vi "Read Menu Queue.vi"(8 "error in (no error)":errorcluster, 11 "Interface with menu in":refnum<class "Interface with menu.lvclass">) -> (0 "error out":errorcluster, 2 "Actor Framework.lvlib:Message Enqueuer":refnum<class "Message Enqueuer.lvclass">, 3 "Interface with menu out":refnum<class "Interface with menu.lvclass">)   [LabVIEW 2015, in "Interface with menu.lvclass"]
uses:
  Interface with menu.lvclass
  <vilib>/ActorFramework/Message Enqueuer/Message Enqueuer.lvclass
  Interface with menu.lvclass/Interface with menu.ctl
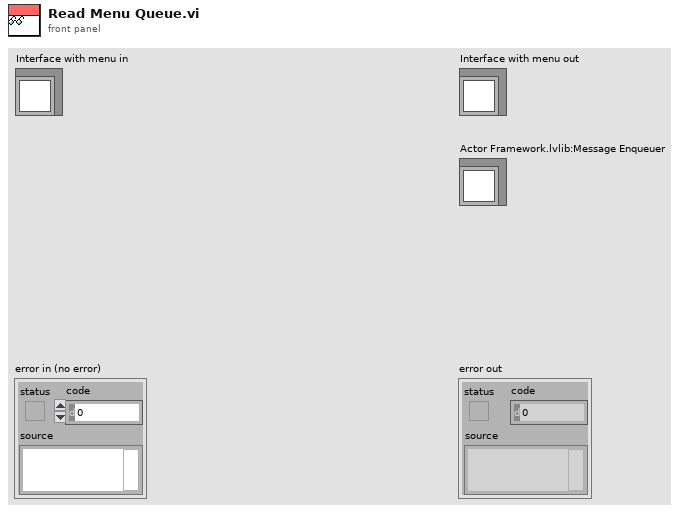
[diagram p1: front panel]
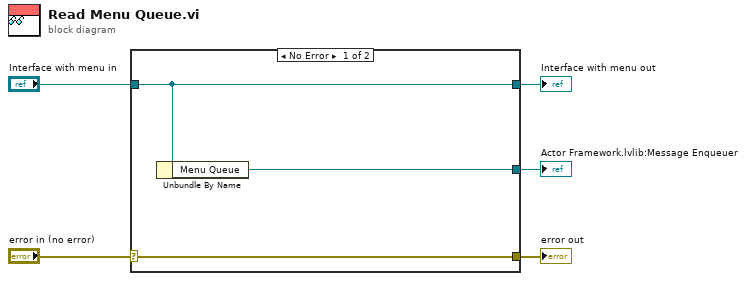
[diagram p0: block diagram]
diagram:
  n1 = case shown="No Error" "error in (no error)" {
    selector: "error in (no error)" -> [w8 w9]
    tunnel: [w8 w9] -> w4
    tunnel: [w7 w10] -> w2
    tunnel: "Interface with menu in" -> [w7 w10]
    tunnel: [w6 _] -> w1
    frame No Error {
      n2 = Unbundle By Name(w7) -> ("Menu Queue"=w6:refnum<class "Message Enqueuer.lvclass">)
    }
    frame Error {
    }
  }
  "error out" <- w4
  "Interface with menu out" <- w2
  "Actor Framework.lvlib:Message Enqueuer" <- w1
